vi "Validate_Destinations.vi"(8 "error in (no error)":errorcluster, 11 "AB_Build in":refnum<class "AB_Build.lvclass">) -> (0 "error out":errorcluster, 3 "AB_Build out":refnum<class "AB_Build.lvclass">)   [LabVIEW 2020, in "AB_Build.lvclass"]
uses:
  <vilib>/AppBuilder/AB_Classes/Build/AB_Build.lvclass
  <vilib>/AppBuilder/AB_Classes/Build/AB_Build.lvclass/AB_Build.ctl
  <vilib>/AppBuilder/AB_Classes/Destination/AB_Destination.ctl
  <resource>/Framework/Providers/Common/provcom_StringGlobals.vi
  <vilib>/AppBuilder/AB_Classes/Destination/AB_Destination.lvclass
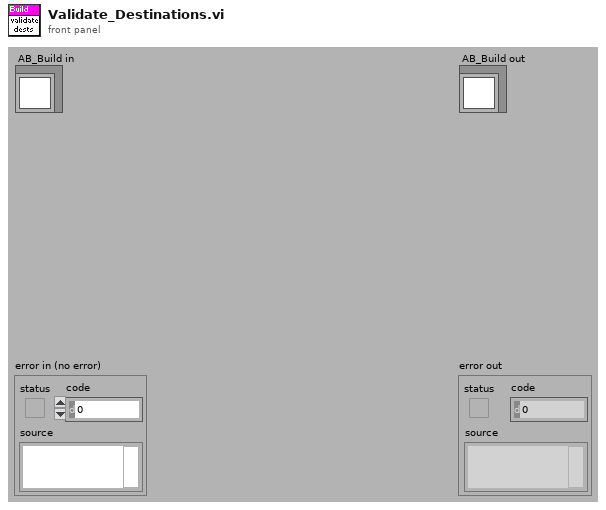
[diagram p1: front panel]
types:
  T1 = typedef "AB_Destination.ctl" = cluster{"destName":string, "path":path, "libraryName":string, "preserveHierarchy":bool, "eng_inBuild":bool, "eng_libraryReference":refnum<vi>, "eng_restictAddToNewLibrary":bool}
  T2 = typedef "ItemRef.ctl" = u64
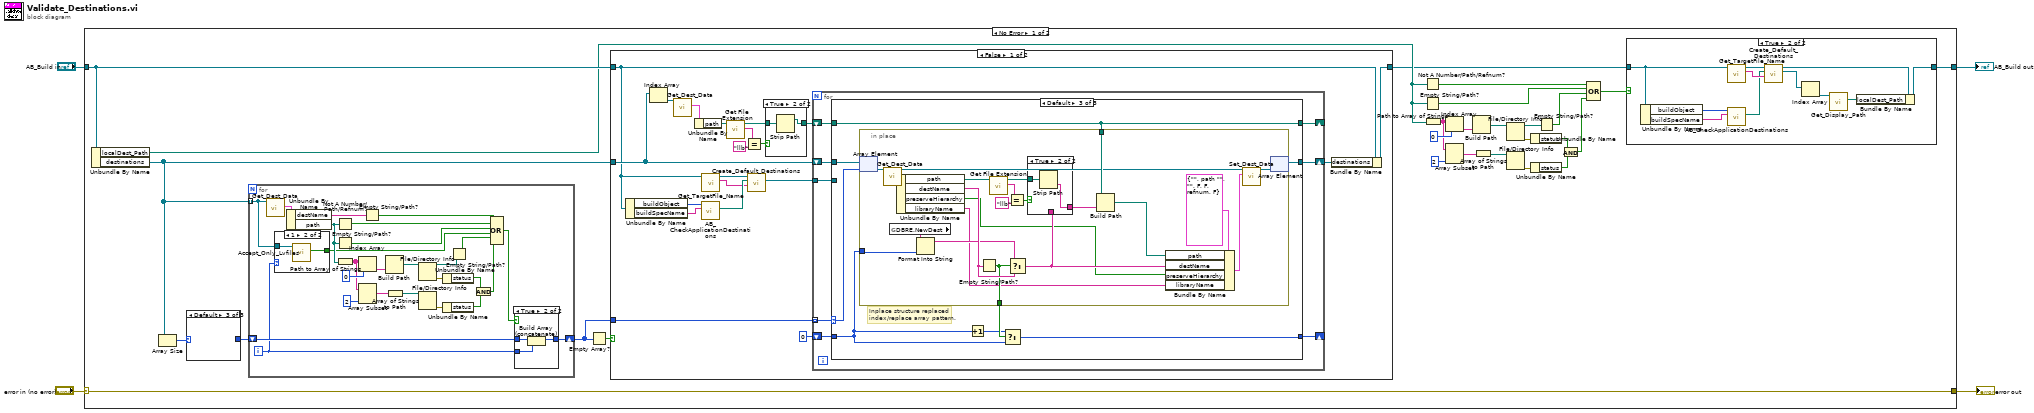
[diagram p0: block diagram]
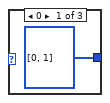
[diagram p3: hidden frame]
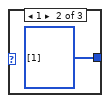
[diagram p4: hidden frame]
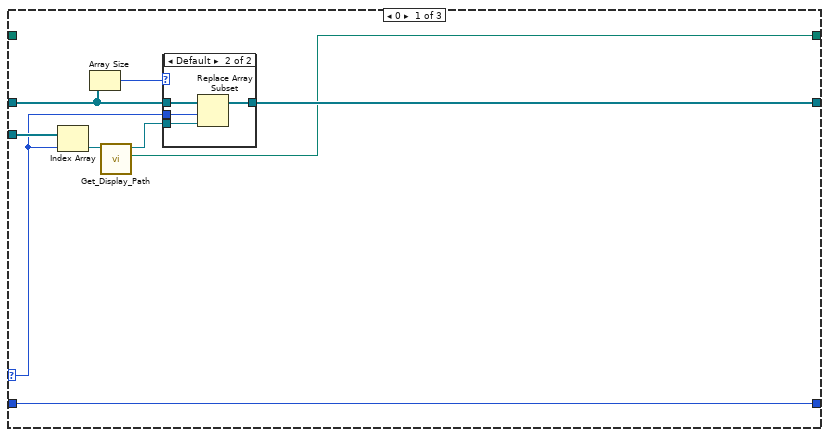
[diagram p5: hidden frame]
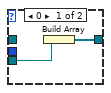
[diagram p6: hidden frame]
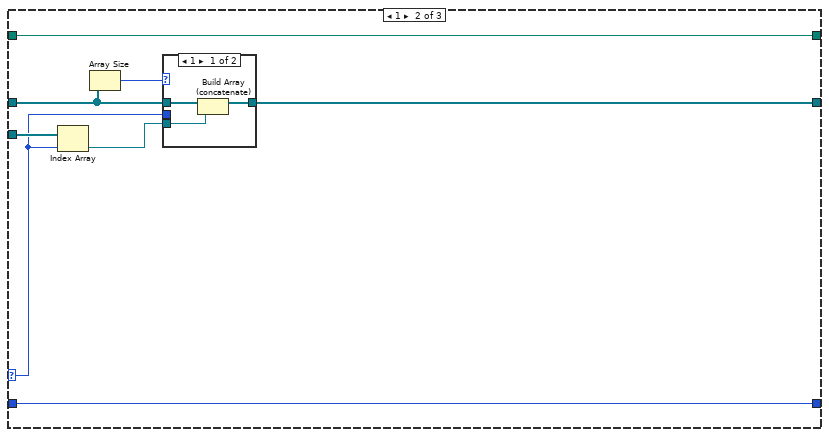
[diagram p7: hidden frame]
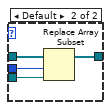
[diagram p8: hidden frame]
diagram:
  n1 = case shown="No Error" "error in (no error)" {
    selector: "error in (no error)" -> [w31 w174]
    tunnel: [w31 w174] -> w3
    tunnel: [w6 w173] -> w1
    tunnel: "AB_Build in" -> [w30 w173]
    frame No Error {
      n2 = Unbundle By Name(w30) -> ("localDest_Path"=w8:path, "destinations"=w27:refnum<class "AB_Destination.lvclass">[])
      n3 = Array Size(array=w27) -> (size(s)=w26:i32)
      n4 = case shown="Default" w26 {
        tunnel: [i32[] [0, 1] i32[] [1] _] -> w25
        frame 0 {
        }
        frame 1 {
        }
        frame Default {
        }
      }
      n5 = for {
        tunnel: w27 -> [w151] mode=indexing
        shift-right: [w156] -> w29
        shift-left: w25 -> [w155]
        i -> [w152]
        n6 = call <vilib>:"Get_Dest_Data.vi"("Class in"=w151) -> ("destName"=w166:T1)  [unwired: 1 in, 9 out]
        n7 = case shown="1" w152 {
          tunnel: w151 -> [_ w168]
          tunnel: [_ w167] -> w150
          frame Default {
          }
          frame 1 {
            n8 = call-dynamic "Accept_Only_Lvfiles.vi"("AB_Destination in"=w168) -> ("onlyLVfiles"=w167:bool)  [unwired: 1 in, 9 out]
          }
        }
        n9 = Unbundle By Name(w166) -> ("destName"=w154:string, "path"=w164:path)
        n10 = Not A Number/Path/Refnum?(number/path/refnum=w164) -> (NaN/Path/Refnum?=w160:bool)
        n11 = Empty String/Path?(string/path=w164) -> (empty?=w159:bool)
        n12 = Path to Array of Strings(0:w164) -> (2:w149:string[])  [unwired: 1 out]
        n13 = Index Array(array=w149, index=0) -> (element=w162:string)
        n14 = Array Subset(array=w149, length=2) -> (w147:string[])  [unwired: 1 in]
        n15 = Empty String/Path?(string/path=w154) -> (empty?=w153:bool)
        n16 = Build Path(name or relative path=w162) -> (appended path=w161:path)  [unwired: 1 out]
        n17 = Array of Strings to Path(0:w147) -> (2:w145:path)  [unwired: 1 out]
        n18 = File/Directory Info(path=w161) -> (path out=w142:path, error out=w165:errorcluster)  [unwired: 1 in, 5 out]
        n19 = File/Directory Info(path=w145) -> (error out=w146:errorcluster)  [unwired: 1 in, 6 out]
        n20 = Unbundle By Name(w165) -> ("status"=w144:bool)
        n21 = Unbundle By Name(w146) -> ("status"=w143:bool)
        n22 = Empty String/Path?(string/path=w142) -> (empty?=w158:bool)
        n23 = And(x=w144, y=w143) -> (x .and. y?=w141:bool)
        n24 = Compound Arithmetic op=OR(w153, w160, w159, w150, w158, w141) -> (w157:bool)
        n25 = case shown="True" w157 {
          tunnel: w152 -> [_ w172]
          tunnel: [w169 w171] -> w156
          tunnel: w155 -> [w169 w170]
          frame False {
          }
          frame True {
            n26 = Build Array (concatenate)(w170, w172) -> (w171:i32[])
          }
        }
      }
      n27 = Empty Array?(array=w29) -> (empty?=w28:bool)
      n28 = case shown="False" w28 {
        tunnel: w29 -> [w65 _]
        tunnel: [w64 w140] -> w7
        tunnel: w30 -> [w48 w140]
        tunnel: w27 -> [w51 _]
        frame False {
          n29 = Unbundle By Name(w48) -> ("buildObject"=w54:T2, "buildSpecName"=w55:string)
          n30 = Index Array(array=w51) -> (element=w59:refnum<class "AB_Destination.lvclass">)  [unwired: 1 in]
          n31 = call <vilib>:"Get_Dest_Data.vi"("Class in"=w59) -> ("destName"=w60:T1)  [unwired: 1 in, 9 out]
          n32 = Unbundle By Name(w60) -> ("path"=w61:path)
          n33 = call <vilib>:"AB_CheckApplicationDestinations.vi"("buildSpecName"=w55, "buildObject"=w54) -> ("Checked base path"=w50:path)  [unwired: 3 in, 6 out]
          n34 = call-dynamic "Get_TargetFile_Name.vi"("Build in"=w48) -> ("targetfile name"=w47:string, "Build out"=w46:refnum<class "AB_Build.lvclass">)  [unwired: 1 in, 8 out]
          n35 = call <vilib>:"Get File Extension.vi"("file"=w61) -> ("lowercase file extension"=w62:string, "dup file"=w58:path)  [unwired: 1 in, 8 out]
          n36 = Equal?(x=w62, y="llb") -> (x = y?=w57:bool)
          n37 = call-dynamic "Create_Default_Destinations.vi"("Destination Name"=w47, "Destination Path"=w50, "AB_Build in"=w46) -> ("default dests"=w49:refnum<class "AB_Destination.lvclass">[])  [unwired: 1 in, 7 out]
          n38 = case shown="True" w57 {
            tunnel: w58 -> [w137 w139]
            tunnel: [w137 w138] -> w56
            frame False {
            }
            frame True {
              n39 = Strip Path(path=w139) -> (stripped path=w138:path)  [unwired: 1 out]
            }
          }
          n40 = for {
            tunnel: w65 -> [w71] mode=indexing
            shift-right: [w73] -> w52
            shift-left: w51 -> [w72]
            shift-right: [w70] -> _
            shift-left: w56 -> [w68]
            tunnel: w49 -> [w69]
            shift-right: [w66] -> _
            shift-left: 0 -> [w67]
            n41 = case shown="Default" w71 {
              selector: w71 -> [w77 w93 w106]
              tunnel: [w82 w96 w104] -> w73
              tunnel: w72 -> [w75 w92 w105]
              tunnel: [w76 w89 w111] -> w70
              tunnel: w69 -> [w81 w95 _]
              tunnel: w68 -> [_ w89 w111]
              tunnel: w67 -> [w78 w94 w107]
              tunnel: [w78 w94 w108] -> w66
              frame 0 {
                n42 = Index Array(array=w81, index=w77) -> (element=w80:refnum<class "AB_Destination.lvclass">)
                n43 = Array Size(array=w75) -> (size(s)=w74:i32)
                n44 = call-dynamic "Get_Display_Path.vi"("AB_Destination in"=w80) -> ("displayPath"=w76:path, "AB_Destination out"=w79:refnum<class "AB_Destination.lvclass">)  [unwired: 1 in, 8 out]
                n45 = case shown="Default" w74 {
                  tunnel: [w83 w88] -> w82
                  tunnel: w75 -> [_ w87]
                  tunnel: w79 -> [w84 w86]
                  tunnel: w77 -> [_ w85]
                  frame 0 {
                    n46 = Build Array(w84) -> (w83:refnum<class "AB_Destination.lvclass">[])
                  }
                  frame Default {
                    n47 = Replace Array Subset(array=w87, new element=w86, index=w85) -> (w88:refnum<class "AB_Destination.lvclass">[])
                  }
                }
              }
              frame 1 {
                n48 = Index Array(array=w95, index=w93) -> (element=w90:refnum<class "AB_Destination.lvclass">)
                n49 = Array Size(array=w92) -> (size(s)=w91:i32)
                n50 = case shown="1" w91 {
                  tunnel: [w98 w103] -> w96
                  tunnel: w92 -> [w97 w102]
                  tunnel: w90 -> [w99 w101]
                  tunnel: w93 -> [_ w100]
                  frame 1 {
                    n51 = Build Array (concatenate)(w97, w99) -> (w98:refnum<class "AB_Destination.lvclass">[])
                  }
                  frame Default {
                    n52 = Replace Array Subset(array=w102, new element=w101, index=w100) -> (w103:refnum<class "AB_Destination.lvclass">[])
                  }
                }
              }
              frame Default {
                # "Inplace structure replaced index/replace array pattern."
                n53 = in-place {
                  in-place-border: w111 -> [w131]
                  in-place-border: [w129] -> w110
                  in-place-border: w107 -> [w125]
                  n54 = in-place-array #1(w105, w106) -> (w123:refnum<class "AB_Destination.lvclass">)
                  n55 = call <vilib>:"Get_Dest_Data.vi"("Class in"=w123) -> ("destName"=w132:T1, "Class out"=w121:refnum<class "AB_Destination.lvclass">)  [unwired: 1 in, 8 out]
                  n56 = global read "provcom_StringGlobals.vi" "DBRE.NewDest"() -> (w126:string)
                  n57 = Unbundle By Name(w132) -> ("path"=w116:path, "destName"=w133:string, "preserveHierarchy"=w113:bool, "libraryName"=w112:string)
                  n58 = Format Into String(initial string=w126, w125) -> (resulting string=w124:string)  [unwired: 2 in, 1 out]
                  n59 = Empty String/Path?(string/path=w133) -> (empty?=w129:bool)
                  n60 = call <vilib>:"Get File Extension.vi"("file"=w116) -> ("lowercase file extension"=w119:string, "dup file"=w118:path)  [unwired: 1 in, 8 out]
                  n61 = Equal?(x=w119, y="llb") -> (x = y?=w117:bool)
                  n62 = Select(t=w124, s=w129, f=w133) -> (s? t:f=w114:string)
                  n63 = case shown="True" w117 {
                    tunnel: w118 -> [_ w136]
                    tunnel: [w134 w135] -> w115
                    tunnel: w114 -> [w134 _]
                    frame False {
                    }
                    frame True {
                      n64 = Strip Path(path=w136) -> (name=w135:string)  [unwired: 1 out]
                    }
                  }
                  n65 = Build Path(base path=w131, name or relative path=w115) -> (appended path=w130:path)
                  n66 = Bundle By Name(cluster=T1 {"destName"="", "path"=path "", "libraryName"="", "preserveHierarchy"=FALSE, "eng_inBuild"=FALSE, "eng_libraryReference"=refnum, "eng_restictAddToNewLibrary"=FALSE} ("destName"), "path"=w130, "destName"=w114, "preserveHierarchy"=w113, "libraryName"=w112) -> (w127:T1)
                  n67 = call <vilib>:"Set_Dest_Data.vi"("destName"=w127, "Class in"=w121) -> ("Class out"=w122:refnum<class "AB_Destination.lvclass">)  [unwired: 1 in, 8 out]
                  n68 = in-place-array #1(w122) -> (w104:refnum<class "AB_Destination.lvclass">[])  [unwired: 1 out]
                }
                n69 = Increment(x=w107) -> (x+1=w109:i32)
                n70 = Select(t=w109, s=w110, f=w107) -> (s? t:f=w108:i32)
              }
            }
          }
          n71 = Bundle By Name(cluster=w48, "destinations"=w52) -> (w64:refnum<class "AB_Build.lvclass">)
        }
        frame True {
        }
      }
      n72 = Not A Number/Path/Refnum?(number/path/refnum=w8) -> (NaN/Path/Refnum?=w20:bool)
      n73 = Empty String/Path?(string/path=w8) -> (empty?=w19:bool)
      n74 = Path to Array of Strings(0:w8) -> (2:w17:string[])  [unwired: 1 out]
      n75 = Index Array(array=w17, index=0) -> (element=w22:string)
      n76 = Array Subset(array=w17, length=2) -> (w15:string[])  [unwired: 1 in]
      n77 = Build Path(name or relative path=w22) -> (appended path=w21:path)  [unwired: 1 out]
      n78 = Array of Strings to Path(0:w15) -> (2:w13:path)  [unwired: 1 out]
      n79 = File/Directory Info(path=w21) -> (path out=w10:path, error out=w24:errorcluster)  [unwired: 1 in, 5 out]
      n80 = File/Directory Info(path=w13) -> (error out=w14:errorcluster)  [unwired: 1 in, 6 out]
      n81 = Unbundle By Name(w24) -> ("status"=w12:bool)
      n82 = Unbundle By Name(w14) -> ("status"=w11:bool)
      n83 = Empty String/Path?(string/path=w10) -> (empty?=w18:bool)
      n84 = And(x=w12, y=w11) -> (x .and. y?=w9:bool)
      n85 = Compound Arithmetic op=OR(w20, w19, w18, w9) -> (w5:bool)
      n86 = case shown="True" w5 {
        tunnel: [w32 w36] -> w6
        tunnel: w7 -> [w32 w34]
        frame False {
        }
        frame True {
          n87 = Unbundle By Name(w34) -> ("buildObject"=w40:T2, "buildSpecName"=w39:string)
          n88 = call <vilib>:"AB_CheckApplicationDestinations.vi"("buildSpecName"=w39, "buildObject"=w40) -> ("Checked base path"=w41:path)  [unwired: 3 in, 6 out]
          n89 = call-dynamic "Get_TargetFile_Name.vi"("Build in"=w34) -> ("targetfile name"=w42:string, "Build out"=w43:refnum<class "AB_Build.lvclass">)  [unwired: 1 in, 8 out]
          n90 = call-dynamic "Create_Default_Destinations.vi"("Destination Name"=w42, "Destination Path"=w41, "AB_Build in"=w43) -> ("default dests"=w38:refnum<class "AB_Destination.lvclass">[], "AB_Build out"=w33:refnum<class "AB_Build.lvclass">)  [unwired: 1 in, 6 out]
          n91 = Index Array(array=w38) -> (element=w37:refnum<class "AB_Destination.lvclass">)  [unwired: 1 in]
          n92 = call-dynamic "Get_Display_Path.vi"("AB_Destination in"=w37) -> ("displayPath"=w35:path)  [unwired: 1 in, 9 out]
          n93 = Bundle By Name(cluster=w33, "localDest_Path"=w35) -> (w36:refnum<class "AB_Build.lvclass">)
        }
      }
    }
    frame Error {
    }
  }
  "error out" <- w3
  "AB_Build out" <- w1
